vi "ALTS-2015 Obtain Test data Result DB Driver.vi"(7 "Option":T2, 8 "error in":errorcluster, 10 "Sensor Name":string, 11 "Station Enum":T1) -> (0 "error out":errorcluster, 3 "data":string[][](array[string]))   [LabVIEW 2013]
uses:
  Controls/ALTS-2015 Obtain Test Data DB Driver Options.ctl
  Controls/ALTS-2015 Station Cluster.ctl
  Controls/ALTS-2015 LV2GBL Options.ctl
  <vilib>/addons/database/Connection.llb/Conn ObjectReference.ctl
  <vilib>/addons/database/Connection.llb/DB Tools Open Connec (Path).vi
  <vilib>/addons/database/Connection.llb/Conn Execute.vi
  <vilib>/addons/database/Recordset.llb/Rec Fetch Recordset Data (R).vi
  <vilib>/addons/database/Recordset.llb/Rec Destroy - Connection.vi
  <vilib>/addons/database/NI_Database_API.lvlib
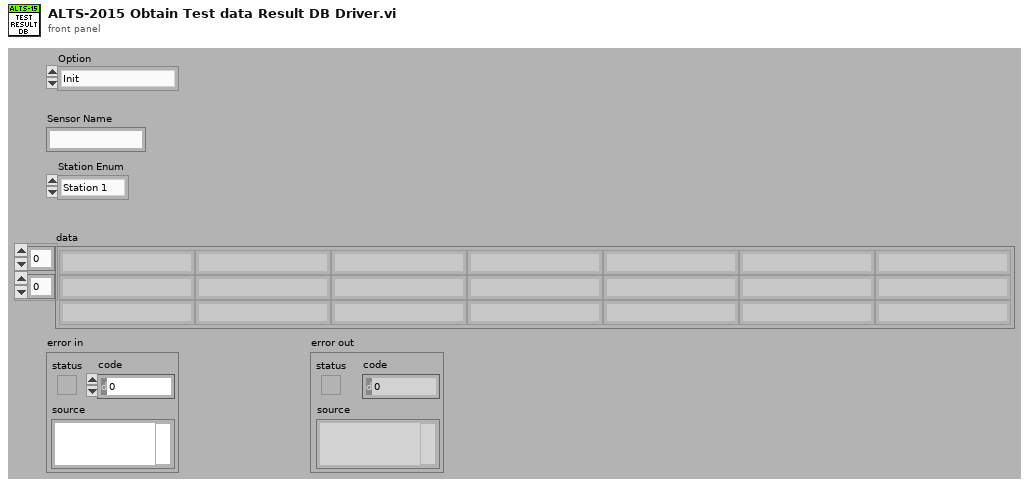
[diagram p1: front panel]
types:
  T1 = typedef "ALTS-2015 Station Cluster.ctl" = enum16{"Station 1", "Station 2", "Station 3", "Station 4"}
  T2 = typedef "ALTS-2015 Obtain Test Data DB Driver Options.ctl" = enum16{"Init", "Read Test Data Results", "Close"}
  T3 = typedef "ALTS-2015 LV2GBL Options.ctl" = enum16{"Read all", "Write all"}
  T4 = typedef "ALTS-2015 INI Configuration Cluster.ctl" = cluster{"Application":cluster{"Rerun Count":i32, "Workorder No":string}, "Station Details":cluster{"Sensor Name 1":string, "Sensor Name 2":string, "Sensor Name 3":string, "Sensor Name 4":string, "Station1 Enable":bool, "Station2 Enable":bool, "Station3 Enable":bool, "Station4 Enable":bool}, "Database":cluster{"Database Connection Link":path, "Result Procedure":string, "User":string, "Password":string, "Prompt":bool, "Station 1 LT Result DB DSN Path":path, "Station 2 LT Result DB DSN Path":path, "Station 3 LT Result DB DSN Path":path, "Station 4 LT Result DB DSN Path":path, "AirLeakTestResult Procedure":string, "Serial Details Procedure":string}, "Simulation":cluster{"Simulate DAQ Hardware":bool, "Simulate Result DB Write":bool, "Simulate Scanner":bool, "Simulate OPC":bool, "Simulate Serial Details DB":bool, "Simulate Result DB":bool, "Simulate Scanner DB Path":path, "Simulate Serial Details DB Path":path, "Simulate Result DB Path":path}, "Barcode Scanner1":cluster{"Scanner IP":string, "Scanner Port":u16, "#Bytes to Read":i32}, "Barcode Scanner2":cluster{"Enabled?":bool, "Scanner IP":string, "Scanner Port":u16, "#Bytes to Read":i32}}
  T5 = typedef "NI_Database_API.lvlib/Conn ObjectReference.ctl" = refnum<k1>
  T6 = typedef "NI_Database_API.lvlib/Rec ObjectReference.ctl" = refnum<k1>
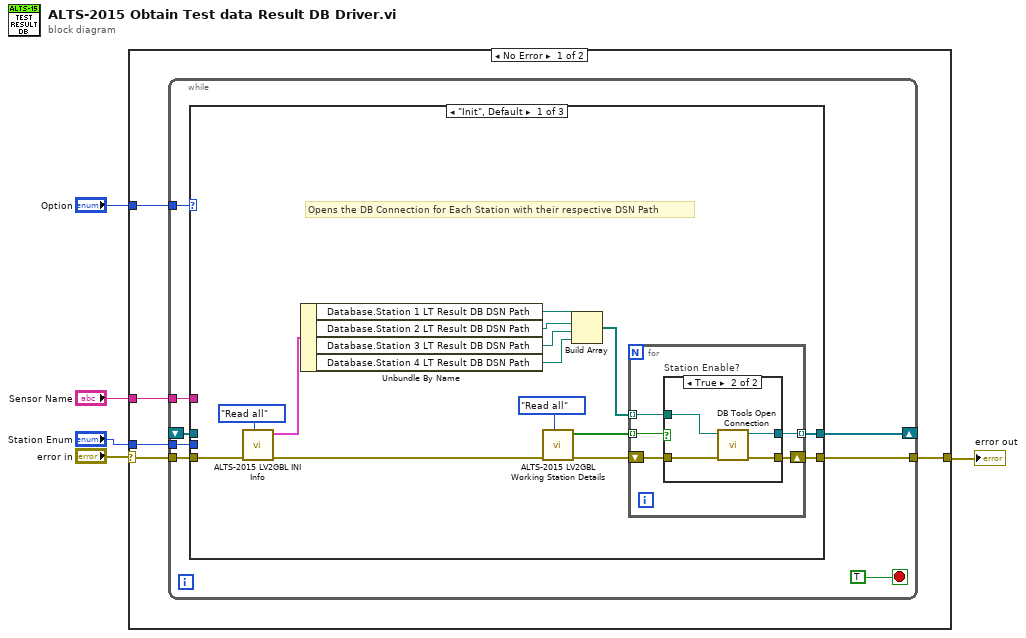
[diagram p0: block diagram]
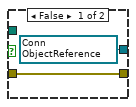
[diagram p2: hidden frame]
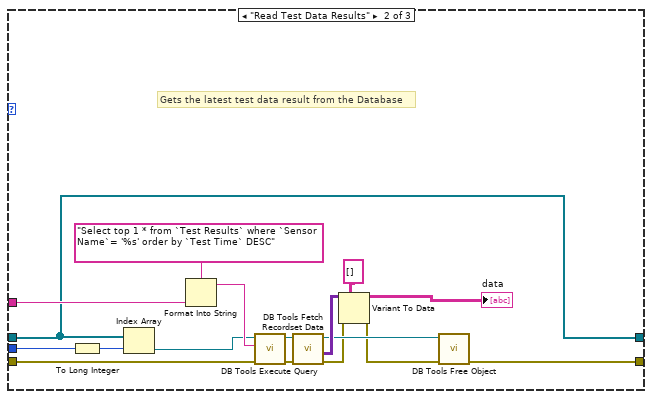
[diagram p3: hidden frame]
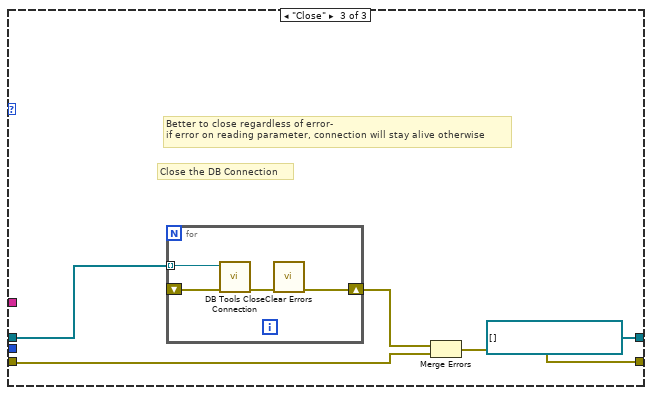
[diagram p4: hidden frame]
diagram:
  n1 = case shown="No Error" "error in" {
    selector: "error in" -> [w10 w70]
    tunnel: [w9 w70] -> w5
    tunnel: "Option" -> [w8 _]
    tunnel: "Sensor Name" -> [w7 _]
    tunnel: "Station Enum" -> [w6 _]
    frame No Error {
      n2 = while {
        tunnel: w10 -> [w17]
        tunnel: [w15] -> w9
        tunnel: w8 -> [w16]
        shift-right: [w12] -> _
        shift-left: _ -> [w14]
        tunnel: w7 -> [w13]
        tunnel: w6 -> [w11]
        stop <- TRUE stop-if-true
        n3 = case shown="\"Init\", Default" w16 {
          tunnel: w17 -> [w32 w52 w63]
          tunnel: [w31 w51 w61] -> w15
          tunnel: w14 -> [_ w47 w65]
          tunnel: w13 -> [_ w48 _]
          tunnel: [w24 w47 w64] -> w12
          tunnel: w11 -> [_ w46 _]
          frame "Init", Default {
            # "Opens the DB Connection for Each Station with their respective DSN Path"
            n4 = call "ALTS-2015 LV2GBL INI Info.vi"("Options"=ALTS-2015_LV2GBL_Options."Read all", "error in"=w32) -> ("error out"=w22:errorcluster, "Configuration Cluster Out"=w30:T4)  [unwired: 8 in]
            n5 = Unbundle By Name(w30) -> ("Database.Station 1 LT Result DB DSN Path"=w29:path, "Database.Station 2 LT Result DB DSN Path"=w28:path, "Database.Station 3 LT Result DB DSN Path"=w27:path, "Database.Station 4 LT Result DB DSN Path"=w26:path)
            n6 = call "ALTS-2015 LV2GBL Working Station Details.vi"("Options"=ALTS-2015_LV2GBL_Options."Read all", "error in"=w22) -> ("error out"=w21:errorcluster, "Station  Enable Array"=w20:bool[])  [unwired: 8 in]
            n7 = Build Array(w29, w28, w27, w26) -> (w25:path[])
            n8 = for {
              tunnel: w25 -> [w36] mode=indexing
              tunnel: [w35] -> w24 mode=indexing
              shift-right: [w37] -> w31
              shift-left: w21 -> [w34]
              tunnel: w20 -> [w33] mode=indexing
              n9 = case "Station Enable?" shown="True" w33 {
                tunnel: [w39 w43] -> w37
                tunnel: w36 -> [_ w42]
                tunnel: [w38 w41] -> w35
                tunnel: w34 -> [w39 w40]
                frame False {
                  w38 = T5 refnum items=["Connection"] ("connection reference")
                }
                frame True {
                  n10 = call-poly <vilib>:"DB Tools Open Connection.vi"("error in (no error)"=w40, "connection information"=w42) -> ("error out"=w43:errorcluster, "connection reference"=w41:T5)  [unwired: 6 in]
                }
              }
            }
          }
          frame "Read Test Data Results" {
            # "Gets the latest test data result from the Database"
            n11 = To Long Integer(number=w46) -> (32bit integer=w45:i32)
            n12 = Index Array(array=w47, index=w45) -> (element=w44:T5)
            n13 = Format Into String(format string="Select top 1 * from `Test Results` where `Sensor Name`= '%s' order by `Test Time` DESC", w48) -> (resulting string=w49:string)  [unwired: 2 in, 1 out]
            n14 = call-poly <vilib>:"DB Tools Execute Query.vi"("error in (no error)"=w52, "SQL query"=w49, "connection reference"=w44) -> ("error out"=w55:errorcluster, "recordset reference"=w54:T6)  [unwired: 5 in]
            n15 = call-poly <vilib>:"DB Tools Fetch Recordset Data.vi"("error in (no error)"=w55, "recordset reference"=w54) -> ("error out"=w57:errorcluster, "recordset data"=w60:variant[][], "recordset reference out"=w59:T6)  [unwired: 3 in]
            n16 = Variant To Data(error in=w57, type=string[][] [], Variant=w60) -> (data=→"data":string[][], error out=w58:errorcluster)
            n17 = call-poly <vilib>:"DB Tools Free Object.vi"("error in (no error)"=w58, "recordset reference"=w59) -> ("error out"=w51:errorcluster)  [unwired: 8 in, 1 out]
          }
          frame "Close" {
            w64 = T5[] [] items=["Connection"]
            # "Better to close regardless of error-\nif error on reading parameter, connection will stay alive otherwise"
            # "Close the DB Connection"
            n18 = for {
              tunnel: w65 -> [w68] mode=indexing
              shift-right: [w66] -> w62
              shift-left: _ -> [w67]
              n19 = call <vilib>:"DB Tools Close Connection.vi"("error in (no error)"=w67, "connection reference"=w68) -> ("error out"=w69:errorcluster)  [unwired: 5 in]
              n20 = call <vilib>:"Clear Errors.vi"("error in (no error)"=w69) -> ("error out"=w66:errorcluster)  [unwired: 6 in]
            }
            n21 = Merge Errors(w62, w63) -> (w61:errorcluster)
          }
        }
      }
    }
    frame Error {
    }
  }
  "error out" <- w5
